vi "BuildBandsList.vi"(9 "Selected Band":string, 11 "Average FRF":cluster{dbl, "df":dbl, dbl[]}[](graph)) -> (1 "Name":string, 2 "updated?":bool)   [LabVIEW 2022 SP3]
uses:
  <vilib>/Utility/error.llb/Trim Whitespace One-Sided.vi
panel:
  in  "Save As":bool
  in  "Save":bool
  in  "delete":bool
  in  "Bands":u16(ring) items=["No Bands", "A Octaves", "Curtin Bands", "JC violin 200-7000 Flat", "JC violin 200-780-1740-2930-7000", "JC violin 200-780-7000", "ObieAlto 200-650-1500-2700-6300"]
  in  "Frequencies":string
  in  "Remove":bool
  in  "Add":bool
  out "Path":path
  out "file names":string[](array[string])
  in  "start":bool
  in  "Cursors":string[][](table)
  in  "OK Button":bool
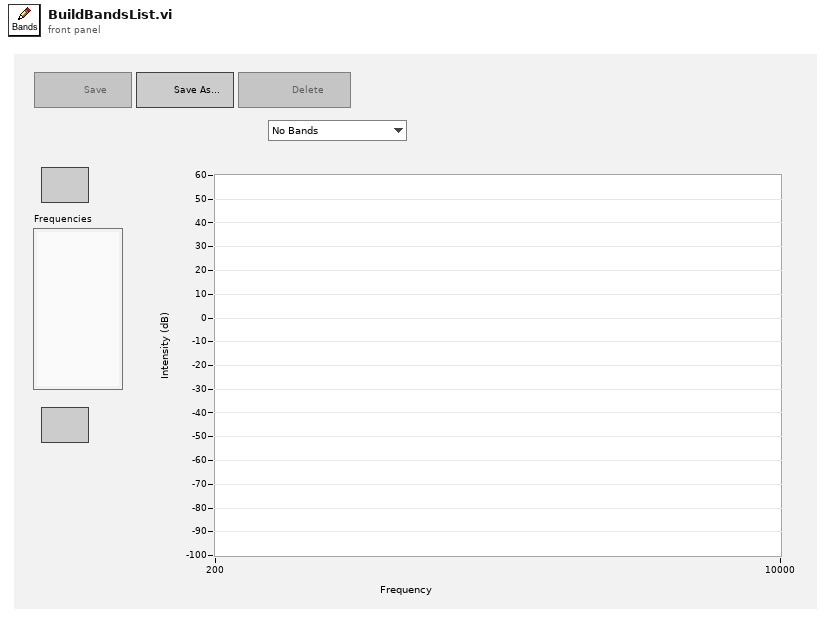
[diagram p1: front panel]
types:
  T1 = enum8{"Enabled", "Disabled", "Disabled and Grayed Out"}
  T2 = typedef "LVCursorListTypeDef.ctl" = cluster{"Name":string, "Color":u32, "Style":u8, "Point Style":u8, "Name Visible":bool, "Allow Drag":bool, "Cursor Mode":u32, "Plot":i32, "Index":i32, "Position":cluster{"X":dbl, "Y":dbl}, "X Scale":u32, "Y Scale":u32, "Watch Plots":i32[], "Watch All Plots":bool, "Plot Area":i32, "Label Offset":cluster{"X":dbl, "Y":dbl}}[]
  T3 = cluster{"Name":string, "Color":u32, "Style":u8, "Point Style":u8, "Name Visible":bool, "Allow Drag":bool, "Cursor Mode":u32, "Plot":i32, "Index":i32, "Position":cluster{"X":dbl, "Y":dbl}, "X Scale":u32, "Y Scale":u32, "Watch Plots":i32[], "Watch All Plots":bool, "Plot Area":i32, "Label Offset":cluster{"X":dbl, "Y":dbl}}[]
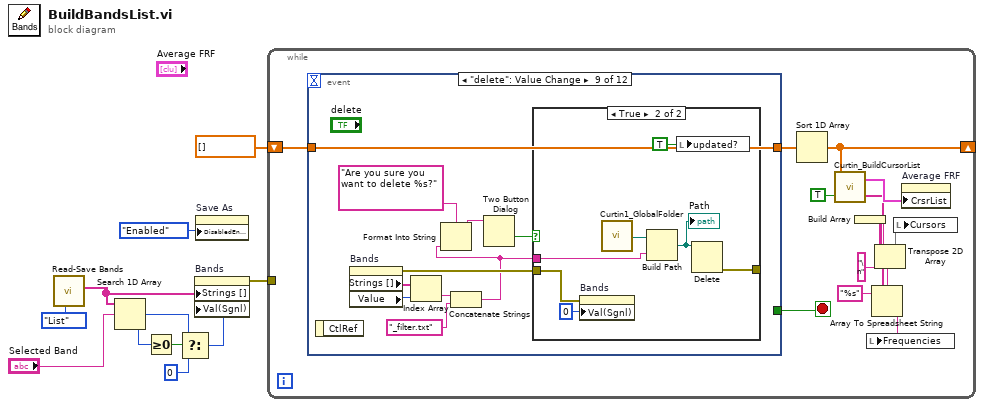
[diagram p0: block diagram]
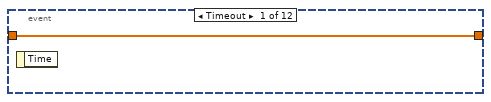
[diagram p2: hidden frame]
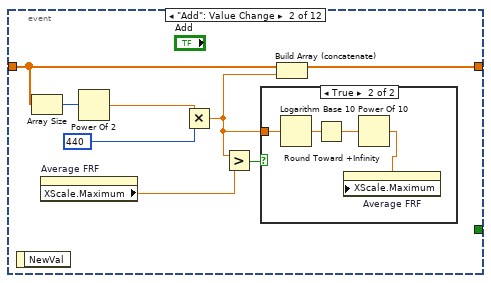
[diagram p3: hidden frame]
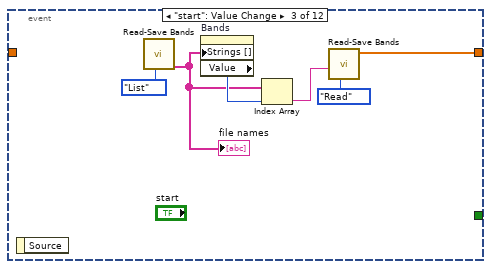
[diagram p5: hidden frame]
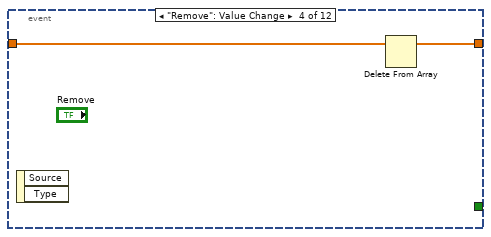
[diagram p6: hidden frame]
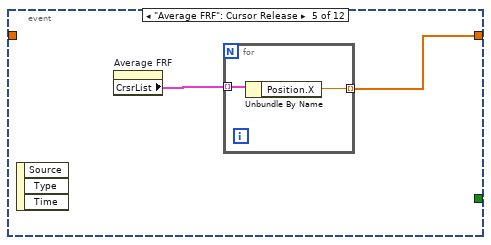
[diagram p7: hidden frame]
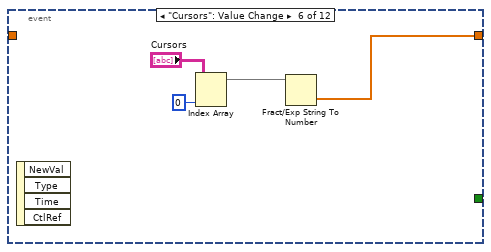
[diagram p8: hidden frame]
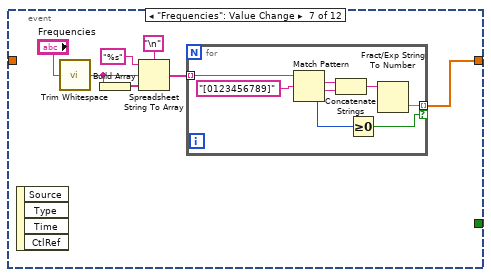
[diagram p9: hidden frame]
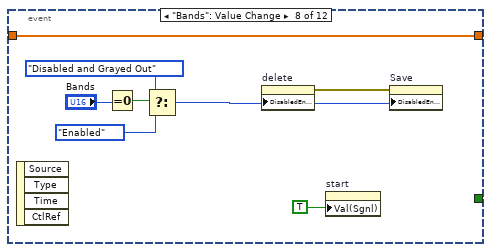
[diagram p10: hidden frame]
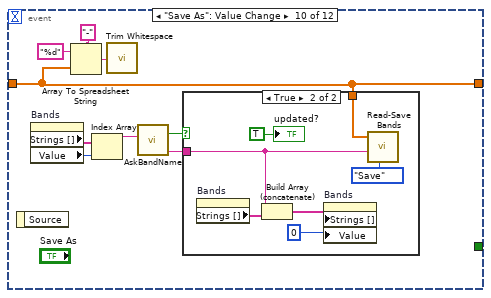
[diagram p12: hidden frame]
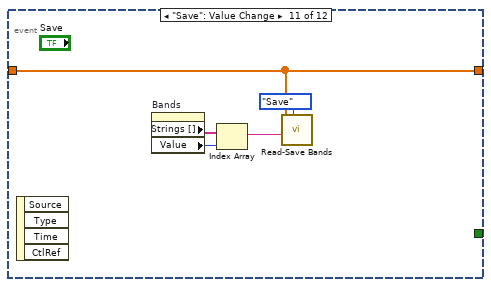
[diagram p14: hidden frame]
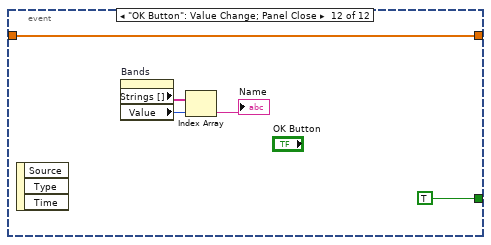
[diagram p15: hidden frame]
diagram:
  n1 = call "Read-Save Bands.vi"("Task"=enum16{"Save", "Read", "List"}."List") -> ("Long names"=w1:string[])  [unwired: 7 in, 3 out]
  n2 = Search 1D Array(1D array=w1, element="Selected Band") -> (index of element=w5:i32)  [unwired: 1 in]
  n3 = Greater Or Equal To 0?(x=w5) -> (x >= 0?=w6:bool)
  n4 = Select(t=w5, s=w6, f=0) -> (s? t:f=w4:i32)
  n5 = property on="Bands" class="Ring (strict)"("Strings []"=w1, "Val(Sgnl)"=w4) -> (error out=w7:errorcluster)  [unwired: 2 in, 1 out]
  n6 = property on="Save As" class="Bool"("DisabledEnum"=T1."Enabled" ("Disabled")) -> ()  [unwired: 2 in, 2 out]
  n7 = while {
    shift-right: [w15] -> _
    shift-left: dbl[] [] -> [w22]
    tunnel: w7 -> [_]
    stop <- w21 stop-if-true
    n8 = event shown="[8] \"delete\": Value Change" {
      selector: _ -> [_ _ _ _ _ _ _ _ _ _ _ _]
      dyn-events: _ -> [_ _ _ _ _ _ _ _ _ _ _ _]
      timeout: _ -> [_ _ _ _ _ _ _ _ _ _ _ _]
      tunnel: w22 -> [w23 w30 _ w43 _ _ _ w70 w84 w92 w111 w116]
      tunnel: [w23 w31 w38 w42 w44 w48 w52 w70 w84 w92 w111 w116] -> w18
      tunnel: [_ _ _ _ _ _ _ _ _ _ _ TRUE ("OK Button")] -> w21
      event Timeout {
        n9 = event-data() -> ()  [unwired: 1 in, 1 out]
      }
      event "Add": Value Change {
        n10 = event-data() -> ()  [unwired: 1 in, 1 out]
        n11 = Array Size(array=w30) -> (size(s)=w29:i32)
        n12 = property on="Average FRF" class="WFGraph (strict)"() -> ("XScale.Maximum"=w26:dbl)  [unwired: 2 in, 2 out]
        n13 = Power Of 2(x=w29) -> (2^x=w28:dbl)
        n14 = Multiply(x=w28, y=440) -> (x*y=w24:dbl)
        n15 = Greater?(x=w24, y=w26) -> (0:w25:bool)
        n16 = case shown="True" w25 {
          tunnel: w24 -> [_ w35]
          frame False {
          }
          frame True {
            n17 = Logarithm Base 10(1:w35) -> (0:w34:dbl)
            n18 = Round Toward +Infinity(x=w34) -> (ceil(x): smallest int >= x=w33:dbl)
            n19 = Power Of 10(x=w33) -> (10^x=w32:dbl)
            n20 = property on="Average FRF" class="WFGraph (strict)"("XScale.Maximum"=w32) -> ()  [unwired: 2 in, 2 out]
          }
        }
        n21 = Build Array (concatenate)(w30, w24) -> (w31:dbl[])
      }
      event "start": Value Change {
        n22 = event-data() -> ()  [unwired: 1 in, 1 out]
        n23 = call "Read-Save Bands.vi"("Task"=enum16{"Save", "Read", "List"}."List") -> ("file names"=w36:string[])  [unwired: 7 in, 3 out]
        "file names" <- w36
        n24 = property on="Bands" class="Ring (strict)"("Strings []"=w36) -> ("Value"=w40:u16)  [unwired: 2 in, 2 out]
        n25 = Index Array(array=w36, index=w40) -> (element=w39:string)
        n26 = call "Read-Save Bands.vi"("Task"=enum16{"Save", "Read", "List"}."Read", "Name"=w39) -> ("Frequencies"=w38:dbl[])  [unwired: 6 in, 3 out]
      }
      event "Remove": Value Change {
        n27 = event-data() -> ()  [unwired: 1 in, 2 out]
        n28 = Delete From Array(array=w43) -> (array with subset deleted=w42:dbl[])  [unwired: 2 in, 1 out]
      }
      event "Average FRF": Cursor Release {
        n29 = event-data() -> ()  [unwired: 1 in, 3 out]
        n30 = property on="Average FRF" class="WFGraph (strict)"() -> ("CrsrList"=w45:T2)  [unwired: 2 in, 2 out]
        n31 = for {
          tunnel: w45 -> [w47] mode=indexing
          tunnel: [w46] -> w44 mode=indexing
          n32 = Unbundle By Name(w47) -> ("Position.X"=w46:dbl)
        }
      }
      event "Cursors": Value Change {
        n33 = event-data() -> ()  [unwired: 1 in, 4 out]
        n34 = Index Array(array="Cursors", index (col)=0 ("disabled index (col)")) -> (element=w49:string[])  [unwired: 1 in]
        n35 = Fract/Exp String To Number(string=w49) -> (number=w48:dbl[])  [unwired: 3 in, 1 out]
      }
      event "Frequencies": Value Change {
        n36 = event-data() -> ()  [unwired: 1 in, 4 out]
        n37 = call <vilib>:"Trim Whitespace.vi"("string"="Frequencies") -> ("trimmed string"=w55:string)  [unwired: 1 in]
        n38 = Build Array(w55) -> (w56:string[])
        n39 = Spreadsheet String To Array(delimiter (Tab)="\n", format string="%s", spreadsheet string=w55, array type (2D Dbl)=w56) -> (array=w54:string[])
        n40 = for {
          tunnel: w54 -> [w66] mode=indexing
          tunnel: [w61] -> w52 mode=indexing if=w59
          n41 = Match Pattern(string=w66, regular expression="[0123456789]") -> (match substring=w64:string, after substring=w63:string, offset past match=w60:i32)  [unwired: 1 in, 1 out]
          n42 = Concatenate Strings(w64, w63) -> (w62:string)
          n43 = Greater Or Equal To 0?(x=w60) -> (x >= 0?=w59:bool)
          n44 = Fract/Exp String To Number(string=w62) -> (number=w61:dbl)  [unwired: 3 in, 1 out]
        }
      }
      event "Bands": Value Change {
        n45 = event-data() -> ()  [unwired: 1 in, 4 out]
        n46 = Equal To 0?(x="Bands") -> (x = 0?=w73:bool)
        n47 = Select(t=T1."Disabled and Grayed Out" ("Disabled"), s=w73, f=T1."Enabled") -> (s? t:f=w68:T1)
        n48 = property on="delete" class="Bool"("DisabledEnum"=w68) -> (error out=w67:errorcluster)  [unwired: 2 in, 1 out]
        n49 = property on="start" class="Bool (strict)"("Val(Sgnl)"=TRUE ("Value (Signaling)")) -> ()  [unwired: 2 in, 2 out]
        n50 = property on="Save" class="Bool"(error in=w67, "DisabledEnum"=w68) -> ()  [unwired: 1 in, 2 out]
      }
      event "delete": Value Change {
        n51 = event-data() -> ()  [unwired: 1 in, 1 out]
        n52 = property on="Bands" class="Ring (strict)"() -> (error out=w77:errorcluster, "Strings []"=w80:string[], "Value"=w79:u16)  [unwired: 2 in, 1 out]
        n53 = Index Array(array=w80, index=w79) -> (element=w81:string)
        n54 = Concatenate Strings(w81, "_filter.txt" ("string")) -> (w76:string)
        n55 = Format Into String(format string="Are you sure you want to delete %s?" ("message"), w76) -> (resulting string=w75:string)  [unwired: 2 in, 1 out]
        n56 = Two Button Dialog(message=w75) -> (T button?=w83:bool)  [unwired: 2 in]
        n57 = case shown="True" w83 {
          tunnel: w77 -> [_ w87]
          tunnel: w76 -> [_ w88]
          tunnel: [_ w86] -> _
          frame False {
          }
          frame True {
            n58 = property on="Bands" class="Ring (strict)"(error in=w87, "Val(Sgnl)"=0 ("index")) -> ()  [unwired: 1 in, 2 out]
            n59 = call "Curtin1_GlobalFolder.vi"() -> ("LabVIEW Data Path"=w89:path)  [unwired: 1 in, 1 out]
            n60 = Build Path(base path=w89, name or relative path=w88) -> (appended path=w85:path)
            "Path" <- w85
            n61 = local write "updated?"(TRUE ("updated?")) -> ()
            n62 = Delete(path (use dialog)=w85) -> (error out=w86:errorcluster)  [unwired: 4 in, 2 out]
          }
        }
      }
      event "Save As": Value Change {
        n63 = event-data() -> ()  [unwired: 1 in, 1 out]
        n64 = property on="Bands" class="Ring (strict)"() -> ("Strings []"=w97:string[], "Value"=w98:u16)  [unwired: 2 in, 2 out]
        n65 = Array To Spreadsheet String(delimiter (Tab)="-", array=w92, 3:"%d" ("format string")) -> (spreadsheet string=w93:string)
        n66 = Index Array(array=w97, index=w98) -> (element=w96:string)
        n67 = call <vilib>:"Trim Whitespace.vi"("string"=w93) -> ()  [unwired: 1 in, 1 out]
        n68 = call "AskBandName.vi"("Default name"=w96) -> ("List"=w99:string, "OK"=w100:bool)  [unwired: 8 in, 1 out]
        n69 = case shown="True" w100 {
          tunnel: w92 -> [_ w107]
          tunnel: w99 -> [_ w102]
          frame False {
          }
          frame True {
            n70 = property on="Bands" class="Ring (strict)"() -> ("Strings []"=w105:string[])  [unwired: 2 in, 2 out]
            n71 = Build Array (concatenate)(w102, w105) -> (w104:string[])
            n72 = property on="Bands" class="Ring (strict)"("Strings []"=w104, "Value"=0) -> ()  [unwired: 2 in, 2 out]
            n73 = call "Read-Save Bands.vi"("Task"=enum16{"Save", "Read"}."Save", "Name"=w102, "Frequencies"=w107) -> ()  [unwired: 5 in, 4 out]
            "updated?" <- TRUE ("updated?")
          }
        }
      }
      event "Save": Value Change {
        n74 = event-data() -> ()  [unwired: 1 in, 4 out]
        n75 = property on="Bands" class="Ring (strict)"() -> ("Strings []"=w109:string[], "Value"=w110:u16)  [unwired: 2 in, 2 out]
        n76 = Index Array(array=w109, index=w110) -> (element=w108:string)
        n77 = call "Read-Save Bands.vi"("Task"=enum16{"Save", "Read"}."Save", "Name"=w108, "Frequencies"=w111) -> ()  [unwired: 5 in, 4 out]
      }
      event "OK Button": Value Change; Panel Close {
        n78 = event-data() -> ()  [unwired: 1 in, 3 out]
        n79 = property on="Bands" class="Ring (strict)"() -> ("Strings []"=w114:string[], "Value"=w115:u16)  [unwired: 2 in, 2 out]
        n80 = Index Array(array=w114, index=w115) -> (element=→"Name":string)
      }
    }
    n81 = Sort 1D Array(array=w18) -> (sorted array=w15:dbl[])
    n82 = call "Curtin_BuildCursorList.vi"("Allow Drag?"=TRUE, "Fctr"=w15) -> ("Freq Titles"=w14:string[], "Cursor List"=w20:T3)
    n83 = Build Array(w14) -> (w17:string[][])
    n84 = Array To Spreadsheet String(delimiter (Tab)="\n", array=w14, 3:"%s" ("format string")) -> (spreadsheet string=w11:string)
    n85 = local write "Frequencies"(w11) -> ()
    n86 = Transpose 2D Array(2D array=w17) -> (transposed array=w16:string[][])
    n87 = local write "Cursors"(w16) -> ()
    n88 = property on="Average FRF" class="WFGraph (strict)"("CrsrList"=w20) -> ()  [unwired: 2 in, 2 out]
  }
